vi "Initialise Address Bus Task.vi"(8 "error in":errorcluster) -> (0 "error out":errorcluster, 3 "Address Bus":refnum<k21> caption="task out")   [LabVIEW 2021, in "IO.lvclass"]
uses:
  IO/IO.lvclass
  <vilib>/DAQmx/create/channels.llb/DAQmx Create Channel (DI-Digital Input).vi
  <resource>/objmgr/daqmx.rc
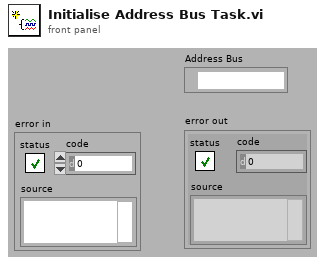
[diagram p1: front panel]
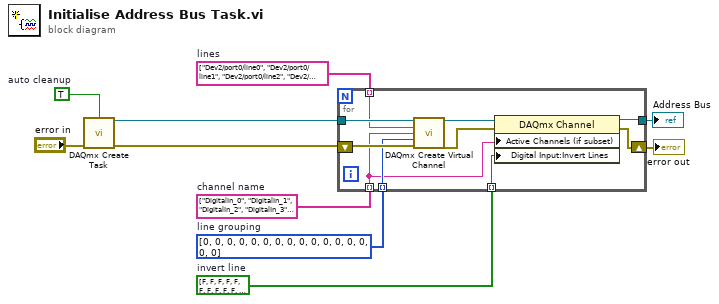
[diagram p0: block diagram]
diagram:
  w6 = bool[] [FALSE, FALSE, FALSE, FALSE, FALSE, FALSE, FALSE, FALSE, FALSE, FALSE, FALSE, FALSE, FALSE, FALSE, FALSE, FALSE]  # invert line
  w5 = i32[] [0, 0, 0, 0, 0, 0, 0, 0, 0, 0, 0, 0, 0, 0, 0, 0] items=["one channel for each line", "one channel for all lines"]  # line grouping
  w4 = string[] ["DigitalIn_0", "DigitalIn_1", "DigitalIn_2", "DigitalIn_3", "DigitalIn_4", "DigitalIn_5", "DigitalIn_6", "DigitalIn_7", "DigitalIn_8", "DigitalIn_9", "DigitalIn_10", "DigitalIn_11", "DigitalIn_12", "DigitalIn_13", "DigitalIn_14", "DigitalIn_15"]  # channel name
  w3 = string[] ["Dev2/port0/line0", "Dev2/port0/line1", "Dev2/port0/line2", "Dev2/port0/line3", "Dev2/port0/line4", "Dev2/port0/line5", "Dev2/port0/line6", "Dev2/port0/line7", "Dev2/port1/line0", "Dev2/port1/line1", "Dev2/port1/line2", "Dev2/port1/line3", "Dev2/port1/line4", "Dev2/port1/line5", "Dev2/port1/line6", "Dev2/port1/line7"]  # lines
  w8 = TRUE  # auto cleanup
  n1 = call <vilib>:"DAQmx Create Task.vi"("auto cleanup"=w8, "error in"="error in") -> ("task out"=w7:refnum<k21>, "error out"=w9:errorcluster)  [unwired: 12 in]
  n2 = for {
    tunnel: w7 -> [w20]
    tunnel: w6 -> [w14] mode=indexing
    tunnel: w5 -> [w17] mode=indexing
    tunnel: w4 -> [w13] mode=indexing
    tunnel: w3 -> [w18] mode=indexing
    tunnel: [w15] -> w2
    shift-right: [w11] -> w1
    shift-left: w9 -> [w19]
    n3 = call-poly <vilib>:"DAQmx Create Virtual Channel.vi"("task in"=w20, "lines"=w18, "name to assign"=w13, "line grouping"=w17, "error in"=w19) -> ("task out"=w16:refnum<k21>, "error out"=w12:errorcluster)  [unwired: 9 in]
    n4 = property class="DAQmx Channel"(reference=w16, error in=w12, "Active Channels (if subset)"=w13, "Digital Input:Invert Lines"=w14) -> (reference out=w15:refnum<k21>, error out=w11:errorcluster)
  }
  "error out" <- w1
  "Address Bus" <- w2
